vi "PKYK_Part_No.vi"(8 "error in (no error)":errorcluster, 10 "table":string, 11 "Refnum in":T1) -> (0 "error out":errorcluster, 2 "PKYK Part Number":string[](array[string]), 3 "Refnum out":T1)   [LabVIEW 2020]
uses:
  <vilib>/addons/database/Connection.llb/Conn ObjectReference.ctl
  <userlib>/_OpenG.lib/array/array.llb/Remove Duplicates from 1D Array (String)__ogtk.vi
  <vilib>/addons/database/_DB Variant To Data/Database Variant To Data.xnode
  <vilib>/addons/database/NI_Database_API.lvlib
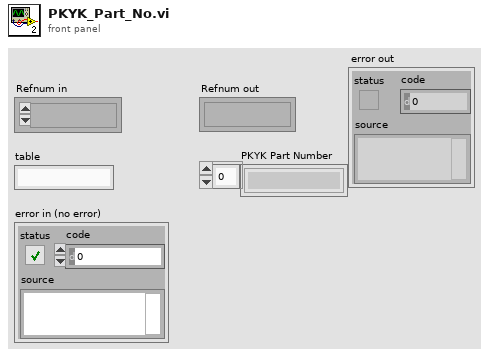
[diagram p1: front panel]
types:
  T1 = typedef "NI_Database_API.lvlib/Conn ObjectReference.ctl" = refnum<k1>
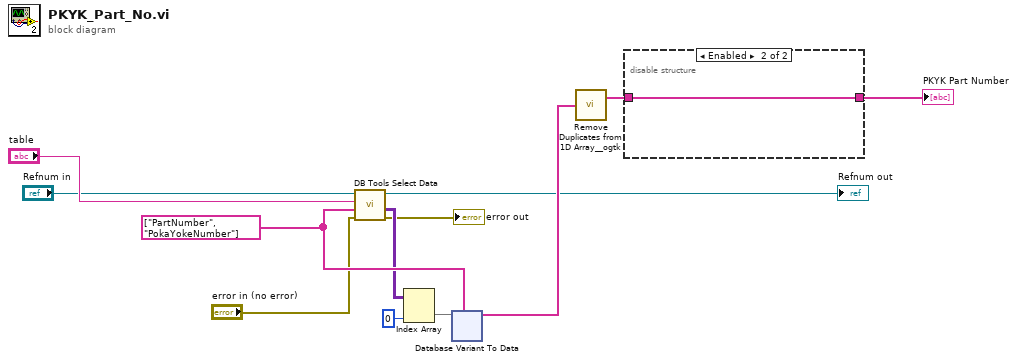
[diagram p0: block diagram]
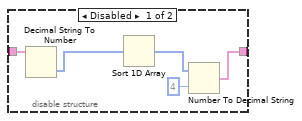
[diagram p2: hidden frame]
diagram:
  w11 = string[] ["PartNumber", "PokaYokeNumber"] ("columns")
  n1 = call <vilib>:"DB Tools Select Data.vi"("error in (no error)"="error in (no error)", "columns"=w11, "table"="table", "connection reference"="Refnum in") -> ("error out"=→"error out":errorcluster, "data"=w5:variant[][], "connection reference out"=→"Refnum out":T1)  [unwired: 2 in]
  n2 = Index Array(array=w5, index (col)=0 ("disabled index (col)")) -> (element=w10:variant[])  [unwired: 1 in]
  n3 = xnode "Database Variant To Data"("database variant"=w10, "type"=w11) -> ("data"=w12:string[])  [unwired: 1 in, 1 out]
  n4 = call-poly <userlib>:"Remove Duplicates from 1D Array__ogtk.vi"("Input Array"=w12) -> ("Output Array"=w2:string[])  [unwired: 1 out]
  n5 = disable-structure shown="Enabled" {
    disable-tunnel: w2 -> [w17 w18]
    disable-tunnel: [w13 w18] -> w1
    frame Disabled {
      n6 = Decimal String To Number(string=w17) -> (number=w16:i32[])  [unwired: 2 in, 1 out]
      n7 = Sort 1D Array(array=w16) -> (sorted array=w15:i32[])
      n8 = Number To Decimal String(number=w15, width (-)=i16 4) -> (decimal integer string=w13:string[])
    }
    frame Enabled {
    }
  }
  "PKYK Part Number" <- w1
